vi "make_while_metadata.vi"(11 "UID":i32) -> (3 "数组":string[](array[string]))   [LabVIEW 2020]
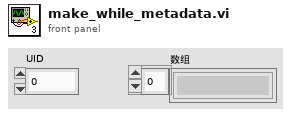
[diagram p1: front panel]
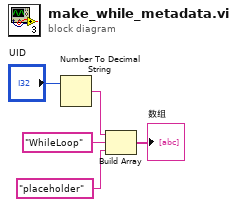
[diagram p0: block diagram]
diagram:
  n1 = Number To Decimal String(number="UID") -> (decimal integer string=w3:string)  [unwired: 1 in]
  n2 = Build Array(w3, "WhileLoop", "placeholder" ("元素")) -> (→"数组":string[])
